vi "example_03_decimation.vi"() -> ()   [LabVIEW 2015, in "lv-graph.lvlib"]
uses:
  _controls/decimation_type.ctl
  advanced/build_graph-single_axis.vi
  lv-graph.lvlib
panel:
  out "data_raw":T1(graph)
  out "data_decimated":T1(graph)
  in  "Data to Generate":i32=100
  in  "Decimation Type":T2
  in  "Decimate Data":bool
  in  "stop":bool
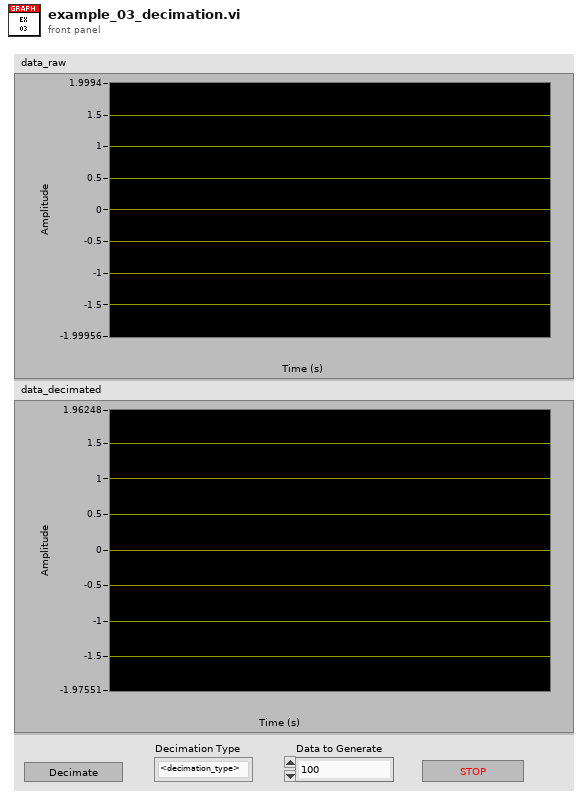
[diagram p1: front panel]
types:
  T1 = cluster{"Time [] out":dbl[], "Data[][] out":dbl[]}[]
  T2 = typedef "lv-graph.lvlib/decimation_type.ctl" = enum16{"<decimation_type>", "average", "min_max", "max", "min", "first", "last"}
  T3 = cluster{"x_scale_maximum":dbl, "x_scale_minimum":dbl, "y_scale_maximum":dbl, "y_scale_minimum":dbl}
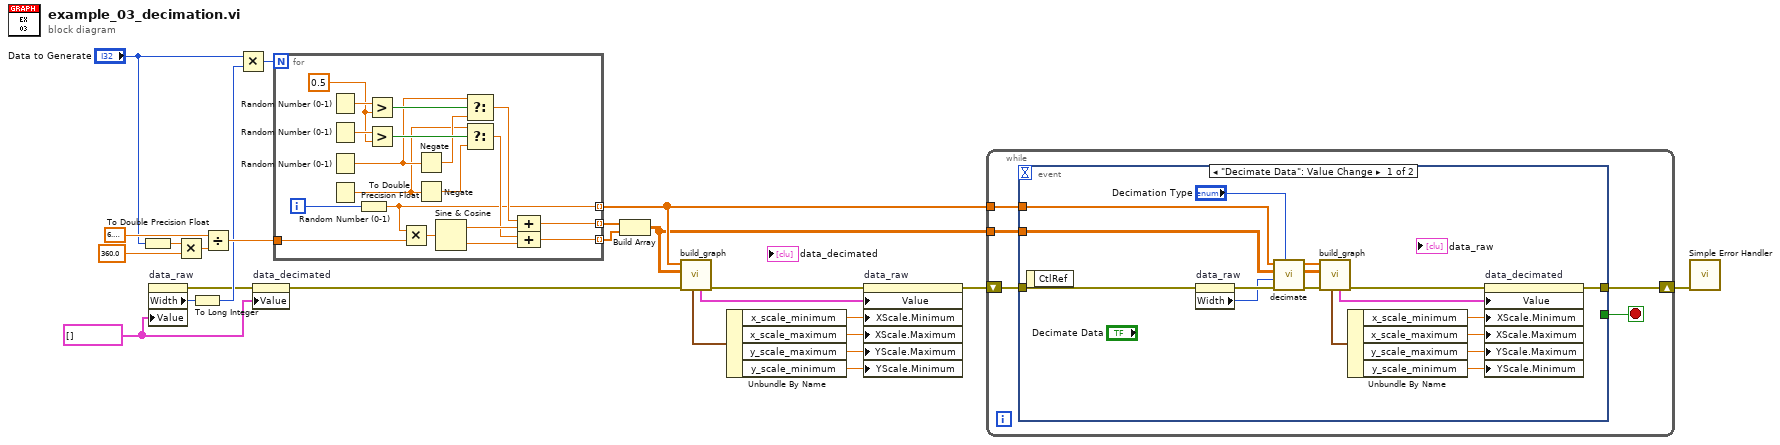
[diagram p0: block diagram]
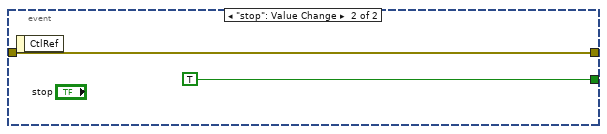
[diagram p2: hidden frame]
diagram:
  w7 = T1 [] ("Graph")
  n1 = To Double Precision Float(number="Data to Generate") -> (double precision float=w11:dbl)
  n2 = property on="data_raw" class="XYGraph (strict)"("Value"=w7) -> (error out=w10:errorcluster, "Width"=w8:u32)  [unwired: 2 in, 1 out]
  n3 = Multiply(x=w11, y=360.0) -> (x*y=w13:dbl)
  n4 = To Long Integer(number=w8) -> (32bit integer=w21:i32)
  n5 = Divide(x=6.283185307179586, y=w13) -> (x/y=w23:dbl)
  n6 = Multiply(x="Data to Generate", y=w21) -> (x*y=w22:i32)
  n7 = property on="data_decimated" class="XYGraph (strict)"(error in=w10, "Value"=w7) -> (error out=w9:errorcluster)  [unwired: 1 in, 1 out]
  n8 = for {
    N: w22 -> [_]
    tunnel: w23 -> [w43]
    tunnel: [w27] -> w6 mode=indexing
    tunnel: [w28] -> w4 mode=indexing
    tunnel: [w26] -> w5 mode=indexing
    i -> [w44]
    w39 = 0.5 ("y")
    n9 = Random Number (0-1)() -> (number: 0 to 1=w41:dbl)
    n10 = Random Number (0-1)() -> (number: 0 to 1=w40:dbl)
    n11 = Random Number (0-1)() -> (number: 0 to 1=w36:dbl)
    n12 = Random Number (0-1)() -> (number: 0 to 1=w34:dbl)
    n13 = To Double Precision Float(number=w44) -> (double precision float=w28:dbl)
    n14 = Greater?(x=w41, y=w39) -> (0:w38:bool)
    n15 = Greater?(x=w40, y=w39) -> (0:w37:bool)
    n16 = Multiply(x=w28, y=w43) -> (x*y=w42:dbl)
    n17 = Negate(x=w36) -> (-x=w35:dbl)
    n18 = Negate(x=w34) -> (-x=w33:dbl)
    n19 = Sine & Cosine(0:w42) -> (1:w31:dbl, 2:w32:dbl)
    n20 = Select(t=w36, s=w38, f=w35) -> (s? t:f=w30:dbl)
    n21 = Select(t=w34, s=w37, f=w33) -> (s? t:f=w29:dbl)
    n22 = Compound Arithmetic op=ADD(w30, w31) -> (w27:dbl)
    n23 = Compound Arithmetic op=ADD(w29, w32) -> (w26:dbl)
  }
  n24 = Build Array(w6, w5) -> (w3:dbl[][])
  n25 = call-poly "build_graph.vi"("error in (no error)"=w9, "y_axis"=w3, "x_axis"=w4) -> ("error out"=w16:errorcluster, "graph_data"=w1:cluster{dbl[], dbl[]}[], "scale_ranges"=w2:T3)  [unwired: 6 in]
  n26 = Unbundle By Name(w2) -> ("x_scale_minimum"=w18:dbl, "x_scale_maximum"=w17:dbl, "y_scale_maximum"=w19:dbl, "y_scale_minimum"=w20:dbl)
  n27 = property on="data_raw" class="XYGraph (strict)"(error in=w16, "Value"=w1, "XScale.Minimum"=w18, "XScale.Maximum"=w17, "YScale.Maximum"=w19, "YScale.Minimum"=w20) -> (error out=w15:errorcluster)  [unwired: 1 in, 1 out]
  n28 = while {
    shift-right: [w47] -> w14
    shift-left: w15 -> [w49]
    tunnel: w4 -> [w46]
    tunnel: w3 -> [w45]
    stop <- w48 stop-if-true
    n29 = event shown="[0] \"Decimate Data\": Value Change" {
      selector: _ -> [_ _]
      dyn-events: _ -> [_ _]
      timeout: _ -> [_ _]
      tunnel: w49 -> [w64 w67]
      tunnel: [_ TRUE] -> w48
      tunnel: [w57 w67] -> w47
      tunnel: w46 -> [w55 _]
      tunnel: w45 -> [w54 _]
      event "Decimate Data": Value Change {
        n30 = event-data() -> ()  [unwired: 1 in, 1 out]
        n31 = property on="data_raw" class="XYGraph (strict)"(error in=w64) -> (error out=w65:errorcluster, "Width"=w56:u32)  [unwired: 1 in, 1 out]
        n32 = call "decimate.vi"("type"="Decimation Type", "error in (no error)"=w65, "height_width"=w56, "y_axis in"=w54, "x_axis in"=w55) -> ("error out"=w63:errorcluster, "y_axis out"=w52:dbl[][], "x_axis out"=w53:dbl[])  [unwired: 4 in]
        n33 = call-poly "build_graph.vi"("error in (no error)"=w63, "y_axis"=w52, "x_axis"=w53) -> ("error out"=w66:errorcluster, "graph_data"=w50:cluster{dbl[], dbl[]}[], "scale_ranges"=w51:T3)  [unwired: 6 in]
        n34 = Unbundle By Name(w51) -> ("x_scale_minimum"=w60:dbl, "x_scale_maximum"=w59:dbl, "y_scale_maximum"=w61:dbl, "y_scale_minimum"=w62:dbl)
        n35 = property on="data_decimated" class="XYGraph (strict)"(error in=w66, "Value"=w50, "XScale.Minimum"=w60, "XScale.Maximum"=w59, "YScale.Maximum"=w61, "YScale.Minimum"=w62) -> (error out=w57:errorcluster)  [unwired: 1 in, 1 out]
      }
      event "stop": Value Change {
        n36 = event-data() -> ()  [unwired: 1 in, 1 out]
      }
    }
  }
  n37 = call <vilib>:"Simple Error Handler.vi"("error in (no error)"=w14) -> ()  [unwired: 4 in, 5 out]
